vi "ACT1.vi"(8 "error in (no error)":errorcluster, 11 "QMH DATA in":refnum<class "QMH DATA.lvclass">) -> (0 "error out":errorcluster, 3 "QMH DATA out":refnum<class "QMH DATA.lvclass">)   [LabVIEW 2020, in "QMH DATA.lvclass"]
uses:
  QMH DATA.lvclass
  QMH DATA.lvclass/QMH DATA.ctl
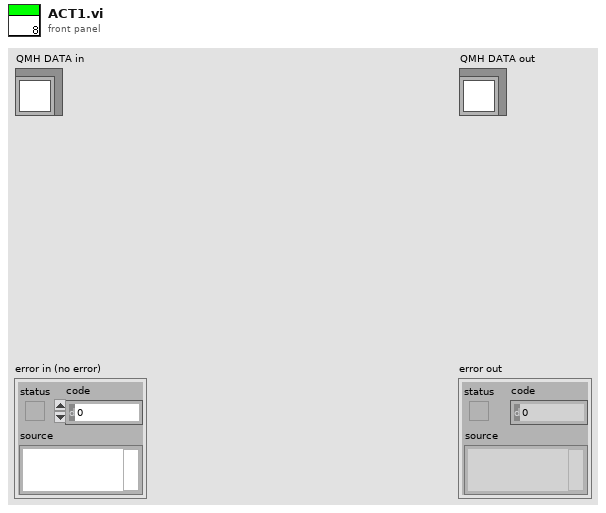
[diagram p1: front panel]
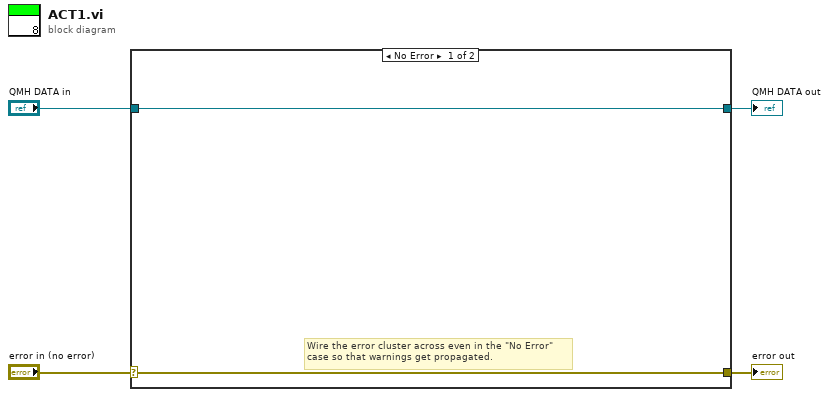
[diagram p0: block diagram]
diagram:
  n1 = case shown="No Error" "error in (no error)" {
    selector: "error in (no error)" -> [w5 w8]
    tunnel: [w5 w8] -> w3
    tunnel: [w6 w7] -> w1
    tunnel: "QMH DATA in" -> [w6 w7]
    frame No Error {
      # "Wire the error cluster across even in the \"No Error\"\ncase so that warnings get propagated."
    }
    frame Error {
    }
  }
  "error out" <- w3
  "QMH DATA out" <- w1
